vi "MKS670_GPIB_set_zero_enable.vi"(7 "mode":enum16{"ON", "OFF"}(ring), 8 "error in":errorcluster, 11 "GPIB in":string) -> (0 "error out":errorcluster, 3 "GPIB out":string, 4 "status":bool)   [LabVIEW 2019]
panel:
  out "comm1":string
  out "string_raw":string
  out "string_fmt":string
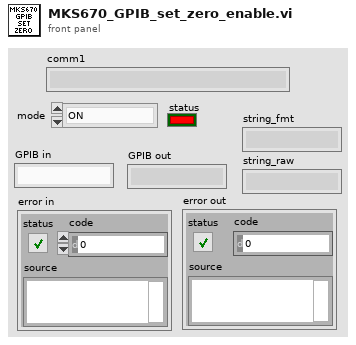
[diagram p1: front panel]
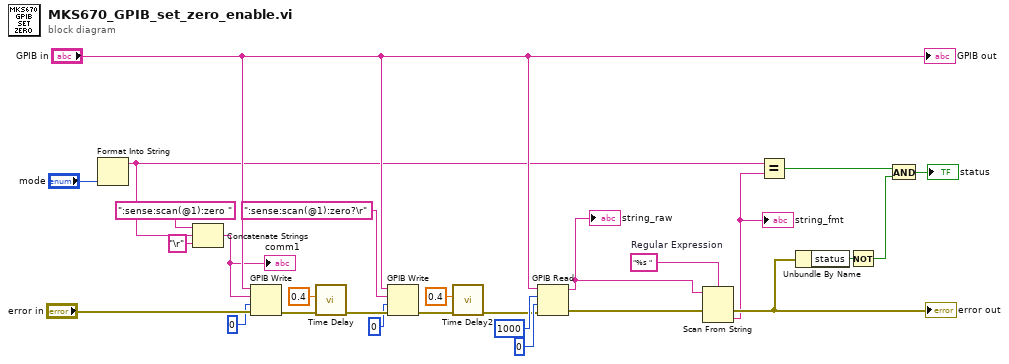
[diagram p0: block diagram]
diagram:
  w25 = "%s "  # Regular Expression
  n1 = Format Into String("mode") -> (resulting string=w2:string)  [unwired: 3 in, 1 out]
  n2 = Concatenate Strings(":sense:scan(@1):zero " ("data"), w2, "\r" ("data")) -> (w4:string)
  "comm1" <- w4
  n3 = GPIB Write(0:"GPIB in", 1:w4, 2:0, 3:"error in") -> (6:w18:errorcluster)  [unwired: 1 in, 1 out]
  n4 = call "Time Delay"("error in (no error)"=w18, "Delay Time (s)"=0.4) -> ("error out"=w14:errorcluster)  [unwired: 9 in]
  n5 = GPIB Write(0:"GPIB in", 1:":sense:scan(@1):zero?\r" ("data"), 2:i16 0 ("mode (0)"), 3:w14) -> (6:w16:errorcluster)  [unwired: 1 in, 1 out]
  n6 = call "Time Delay2"("error in (no error)"=w16, "Delay Time (s)"=0.4) -> ("error out"=w13:errorcluster)  [unwired: 9 in]
  n7 = GPIB Read(0:"GPIB in", 1:1000 ("byte count"), 2:0, 3:w13) -> (5:w24:string, 7:w23:errorcluster)  [unwired: 1 in, 1 out]
  "string_raw" <- w24
  n8 = Scan From String(format string=w25, input string=w24, error in=w23) -> (error out=w22:errorcluster, output 1=w8:string)  [unwired: 2 in, 2 out]
  "string_fmt" <- w8
  "error out" <- w22
  n9 = Equal?(x=w2, y=w8) -> (x = y?=w7:bool)
  n10 = Unbundle By Name(w22) -> ("status"=w20:bool)
  n11 = Not(x=w20) -> (.not. x?=w6:bool)
  n12 = And(x=w7, y=w6) -> (x .and. y?=→"status":bool)
  "GPIB out" <- "GPIB in"
